vi "Begin.vi"() -> (0 "error out":errorcluster)   [LabVIEW 2013]
doc: "Called before other user functions, this VI is expected to open initial I/O refnums, load in file data, and do all program initialization. Notice that the <B>error out</B> terminal is simply used for data flow. Wiring it to other structures or subVIs ensures that this VI runs first."
uses:
  <vilib>/Rock Robotics/WPI/Joystick/WPI_JoystickDeviceEnum.ctl
  <vilib>/Rock Robotics/SystemInterfaces/Typedef/FPGA_TypedefDigitalModule.ctl
  <vilib>/Rock Robotics/SystemInterfaces/DIO/FPGA_DIOChannel.ctl
  <vilib>/Rock Robotics/SystemInterfaces/DIO/FPGA_DIORelayChannel.ctl
  <vilib>/Rock Robotics/SystemInterfaces/Typedef/FPGA_TypedefSolenoidModule.ctl
  <vilib>/Rock Robotics/WPI/Solenoid/WPI_SolenoidChannel.ctl
  <vilib>/Rock Robotics/SystemInterfaces/DIO/FPGA_DIOPWMChannel.ctl
  <vilib>/Rock Robotics/WPI/Encoder/WPI_EncoderType.ctl
  <vilib>/Rock Robotics/WPI/Solenoid/WPI_SolenoidValue.ctl
  <vilib>/Rock Robotics/SystemInterfaces/Typedef/FPGA_TypedefAnalogModule.ctl
  <vilib>/Rock Robotics/SystemInterfaces/AI/FPGA_AIChannel.ctl
  <vilib>/Rock Robotics/WPI/Solenoid/WPI_SolenoidOpenDouble.vi
  <vilib>/Rock Robotics/WPI/Solenoid/WPI_SolenoidSetEnum.vi
  <vilib>/Rock Robotics/WPI/Counter/WPI_CounterDigitalInputToDigitalSource.vi
  <vilib>/Rock Robotics/WPI/MotorControl/WPI_MotorControlOpen Jaguar.vi
  <vilib>/Rock Robotics/WPI/MotorControl/WPI_MotorControlOpen Victor.vi
  <vilib>/Rock Robotics/WPI/RobotDrive/WPI_RobotDriveOpen2MotorWithVictor.vi
  <vilib>/Rock Robotics/WPI/Compressor/WPI_CompressorGetSetRefNum.vi
  <vilib>/Rock Robotics/WPI/Camera/WPI_CameraImageSize.ctl
  <vilib>/Rock Robotics/WPI/Camera/WPI_CameraWhite Balance Values.ctl
  <vilib>/Rock Robotics/WPI/Camera/WPI_CameraExposure Values.ctl
  <vilib>/Rock Robotics/WPI/Camera/WPI_CameraFrameRate.ctl
  <vilib>/Rock Robotics/WPI/RobotDrive/WPI_RobotDriveOpen4MotorWithVictor.vi
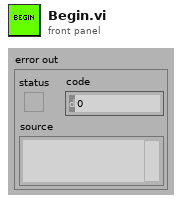
[diagram p1: front panel]
types:
  T1 = typedef "WPI_SolenoidValue.ctl" = enum16{"Off", "On", "Forward", "Reverse"}
  T2 = typedef "FPGA_AIChannel.ctl" = enum8{"AI 1", "AI 2", "AI 3", "AI 4", "AI 5", "AI 6", "AI 7", "AI 8", "Invalid"}
  T3 = typedef "FPGA_TypedefAnalogModule.ctl" = enum16{"Analog Module 1", "Analog Module 2"}
  T4 = typedef "FPGA_DIOChannel.ctl" = enum8{"DIO 1", "DIO 2", "DIO 3", "DIO 4", "DIO 5", "DIO 6", "DIO 7", "DIO 8", "DIO 9", "DIO 10", "DIO 11", "DIO 12", "DIO 13", "DIO 14", "Invalid"}
  T5 = typedef "WPI_SolenoidChannel.ctl" = enum8{"Solenoid 1", "Solenoid 2", "Solenoid 3", "Solenoid 4", "Solenoid 5", "Solenoid 6", "Solenoid 7", "Solenoid 8", "Invalid"}
  T6 = typedef "FPGA_DIOPWMChannel.ctl" = enum8{"PWM 1", "PWM 2", "PWM 3", "PWM 4", "PWM 5", "PWM 6", "PWM 7", "PWM 8", "PWM 9", "PWM 10", "Invalid"}
  T7 = typedef "WPI_EncoderType.ctl" = enum16{"1x", "2x", "4x"}
  T8 = typedef "FPGA_TypedefSolenoidModule.ctl" = enum16{"Solenoid Module 1", "Solenoid Module 2"}
  T9 = typedef "FPGA_DIORelayChannel.ctl" = enum8{"Relay 1", "Relay 2", "Relay 3", "Relay 4", "Relay 5", "Relay 6", "Relay 7", "Relay 8", "Invalid"}
  T10 = typedef "WPI_JoystickDeviceEnum.ctl" = enum16{"USB 1", "USB 2", "USB 3", "USB 4", "Kinect 1", "Kinect 2"}
  T11 = typedef "FPGA_TypedefDigitalModule.ctl" = enum16{"Digital Module 1", "Digital Module 2"}
  T12 = typedef "WPI_CameraFrameRate.ctl" = u32
  T13 = typedef "WPI_CameraExposure Values.ctl" = enum16{"Auto", "Flicker-free 50 Hz", "Flicker-free 60 Hz", "Hold current"}
  T14 = typedef "WPI_CameraWhite Balance Values.ctl" = enum16{"Auto", "Fixed indoor", "Fixed outdoor 1", "Fixed outdoor 2", "Fixed fluorescent 1", "Fixed fluorescent 2", "Hold current"}
  T15 = typedef "WPI_CameraImageSize.ctl" = enum16{"640x480", "320x240", "160x120"}
  T16 = typedef "WPI_CameraDevRef.ctl" = cluster{"Camera Address":string, "CameraStatus":errorcluster, "Acquire Image Notifier":refnum<notifier>}
  T17 = typedef "WPI_DigitalInputDevRef.ctl" = cluster{"DevStatus":errorcluster, "DIO Channel":T4, "Digital Module":T11}
  T18 = typedef "WPI_AnalogChannelDevRef.ctl" = cluster{"DevStatus":errorcluster, "Analog Module":T3, "Analog Channel":T2}
  T19 = typedef "WPI_RobotDriveDevRef.ctl" = cluster{"DevStatus":errorcluster, "Motors[]":T20[], "Square Inputs":bool, "Max Output":dbl, "Isochronous":bool}
  T20 = typedef "WPI_MotorControlDeviceRef.ctl" = cluster{"DeviceStatus":errorcluster, "Type":enum16{"PWM", "CAN"}, "PWM":cluster{"Digital Module":T11, "PWM Channel":T6, "DeadBand":T21}, "CAN":cluster{"Device Number":u8, "Control Mode":T22, "Semaphore":T23, "Max Vout":dbl}, "Invert":bool, "TransformRef":T24, "InvTransformRef":T24}
  T21 = typedef "WPI_PWMDeadband.ctl" = cluster{"Name":string, "maxPositivePwm":i32, "minPositivePwm":i32, "centerPwm":i32, "maxNegativePwm":i32, "minNegativePwm":i32, "angularRange":u16}
  T22 = typedef "WPI_CANJaguar_ControlMode.ctl" = enum8{"Percent VBus", "Current", "Speed", "Position", "Voltage"}
  T23 = typedef "Semaphore RefNum" = refnum<k1>
  T24 = typedef "WPI_PWMTransform_ConPane.ctl" = refnum<vi>
  T25 = typedef "WPI_SolenoidDevRef.ctl" = cluster{"DevStatus":errorcluster, "Solenoid Module":T8, "Forward Solenoid Channel":T5, "Reverse Solenoid Channel":T5}
  T26 = typedef "FPGA_CounterEncoderSourceConvertionLVSourceType.ctl" = cluster{"DevStatus":errorcluster, "AnalogTriggerMode?":bool, "DigitalMode":cluster{"Digital Module":T11, "DIO Channel":T27}, "AnalogTriggerMode":cluster{"AnalogTriggerIndex":T28, "OutputType":T29}}
  T27 = typedef "FPGA_DIODigitalSourceChannel.ctl" = enum8{"DIO 1", "DIO 2", "DIO 3", "DIO 4", "DIO 5", "DIO 6", "DIO 7", "DIO 8", "DIO 9", "DIO 10", "DIO 11", "DIO 12", "DIO 13", "DIO 14", "Disabled"}
  T28 = typedef "FPGA_AnalogTriggerIndex.ctl" = enum8{"Trig 0", "Trig 1", "Trig 2", "Trig 3", "Trig 4", "Trig 5", "Trig 6", "Trig 7", "Invalid"}
  T29 = typedef "FPGA_AnalogTriggerOutType.ctl" = enum16{"InWindow", "TriggerState", "Rising", "Falling"}
  T30 = typedef "WPI_CompressorDevRef.ctl" = cluster{"DevStatus":errorcluster, "DigitalInputDevRef":T17, "RelayDevRef":T31}
  T31 = typedef "WPI_RelayDevRef.ctl" = cluster{"DevStatus":errorcluster, "Relay Channel":T9, "Digital Module":T11, "Relay Direction":T32}
  T32 = typedef "WPI_RelayDirection.ctl" = enum16{"Both directions", "Forward only", "Reverse only"}
  T33 = typedef "WPI_EncoderDevRef.ctl" = cluster{"DevStatus":errorcluster, "EncoderIndex":T34, "CounterIndex":T35, "DistancePerCount":dbl, "Decoding Type":T7}
  T34 = typedef "FPGA_EncoderIdx.ctl" = enum8{"Enc 0", "Enc 1", "Enc 2", "Enc 3", "Invalid"}
  T35 = typedef "FPGA_CounterCtrSystemIndex.ctl" = enum8{"Ctr 0", "Ctr 1", "Ctr 2", "Ctr 3", "Ctr 4", "Ctr 5", "Ctr 6", "Ctr 7", "Invalid"}
  T36 = typedef "WPI_JoystickDevRef.ctl" = cluster{"Device":T10}
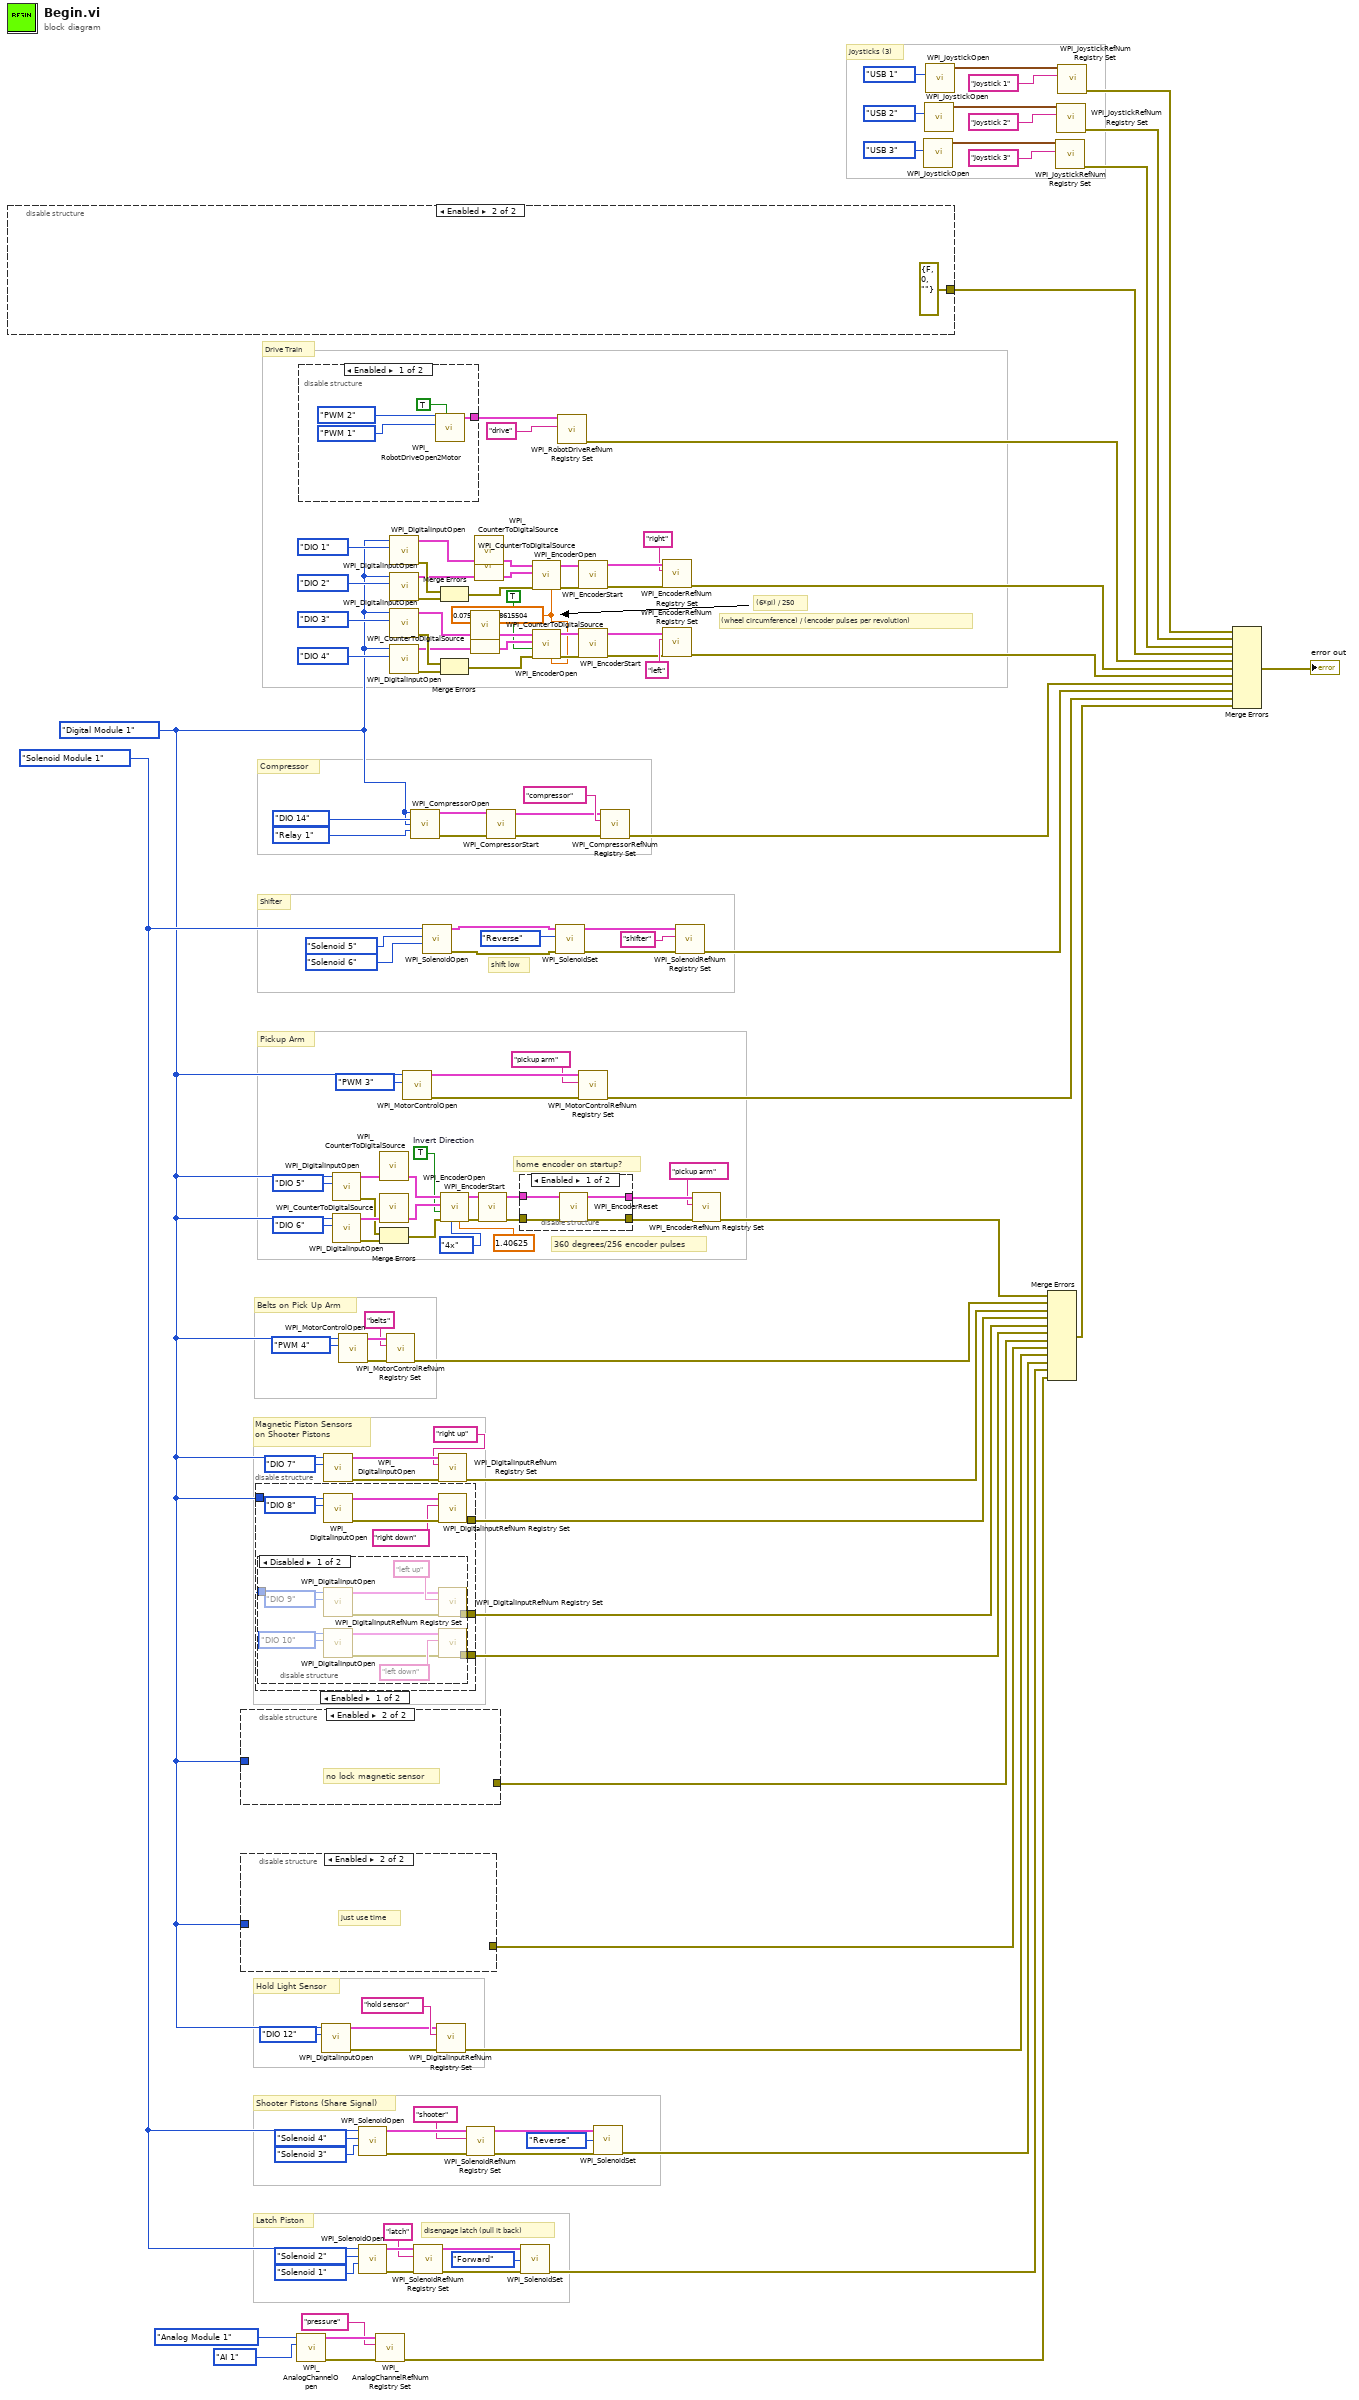
[diagram p0: block diagram]
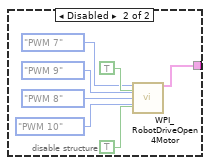
[diagram p2: hidden frame]
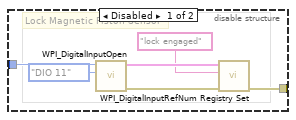
[diagram p3: hidden frame]
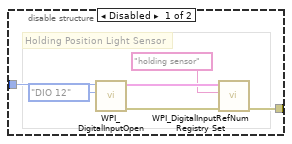
[diagram p6: hidden frame]
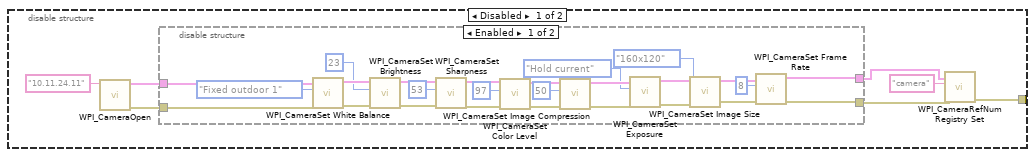
[diagram p8: hidden frame]
diagram:
  w13 = TRUE  # Invert Direction
  w84 = 0.07539822368615504 ("DistancePerCount")
  w27 = FPGA_TypedefSolenoidModule."Solenoid Module 1" ("Solenoid Module (Module 1)")
  w20 = FPGA_TypedefDigitalModule."Digital Module 1" ("Digital Module (Module 1)")
  # "360 degrees/256 encoder pulses"
  # "disengage latch (pull it back)"
  # "Hold Light Sensor"
  # "Joysticks (3)"
  # "Latch Piston"
  # "Shooter Pistons (Share Signal)"
  # "Magnetic Piston Sensors\non Shooter Pistons"
  # "Belts on Pick Up Arm"
  # "Pickup Arm"
  # "home encoder on startup?"
  # "Shifter"
  # "Compressor"
  # "Drive Train"
  # "shift low"
  # "(wheel circumference) / (encoder pulses per revolution)"
  # "(6*pi) / 250"
  n1 = disable-structure shown="Enabled" {
    disable-tunnel: [w139 errorcluster {"status"=FALSE, "code"=0, "source"=""} ("error out")] -> w126
    frame Disabled {
      n2 = call <vilib>:"WPI_CameraOpen.vi"("Camera Address"="10.11.24.11") -> ("error out"=w141:errorcluster, "CameraDevRef"=w143:T16)  [unwired: 9 in]
      n3 = disable-structure shown="Enabled" {
        disable-tunnel: w143 -> [w169 w173]
        disable-tunnel: [w147 w173] -> w142
        disable-tunnel: w141 -> [w156 w172]
        disable-tunnel: [w146 w172] -> w140
        frame Enabled {
          n4 = call <vilib>:"WPI_CameraSet White Balance.vi"("error in (no error)"=w156, "White Balance"=WPI_CameraWhite_Balance_Values."Fixed outdoor 1", "CameraDevRef"=w169) -> ("error out"=w157:errorcluster, "CameraDevRef Out"=w168:T16)  [unwired: 7 in]
          n5 = call <vilib>:"WPI_CameraSet Brightness.vi"("error in (no error)"=w157, "Brightness"=23, "CameraDevRef"=w168) -> ("error out"=w158:errorcluster, "CameraDevRef Out"=w167:T16)  [unwired: 7 in]
          n6 = call <vilib>:"WPI_CameraSet Sharpness.vi"("error in (no error)"=w158, "Sharpness"=53, "CameraDevRef"=w167) -> ("error out"=w159:errorcluster, "CameraDevRef Out"=w166:T16)  [unwired: 7 in]
          n7 = call <vilib>:"WPI_CameraSet Color Level.vi"("error in (no error)"=w159, "Color Level"=97, "CameraDevRef"=w166) -> ("error out"=w160:errorcluster, "CameraDevRef Out"=w165:T16)  [unwired: 7 in]
          n8 = call <vilib>:"WPI_CameraSet Image Compression.vi"("error in (no error)"=w160, "Compression"=50, "CameraDevRef"=w165) -> ("error out"=w171:errorcluster, "CameraDevRef Out"=w170:T16)  [unwired: 7 in]
          n9 = call <vilib>:"WPI_CameraSet Exposure.vi"("error in (no error)"=w171, "Exposure"=WPI_CameraExposure_Values."Hold current", "CameraDevRef"=w170) -> ("error out"=w161:errorcluster, "CameraDevRef Out"=w164:T16)  [unwired: 7 in]
          n10 = call <vilib>:"WPI_CameraSet Image Size.vi"("error in (no error)"=w161, "Image Size"=WPI_CameraImageSize."160x120", "CameraDevRef"=w164) -> ("error out"=w162:errorcluster, "CameraDevRef Out"=w163:T16)  [unwired: 7 in]
          n11 = call <vilib>:"WPI_CameraSet Frame Rate.vi"("error in (no error)"=w162, "Frame Rate (fps)"=T12 8, "CameraDevRef"=w163) -> ("error out"=w146:errorcluster, "CameraDevRef Out"=w147:T16)  [unwired: 7 in]
        }
        frame Disabled {
        }
      }
      n12 = call <vilib>:"WPI_CameraRefNum Registry Set.vi"("error in (no error)"=w140, "refnum name"="camera", "CameraDevRef"=w142) -> ("error out"=w139:errorcluster)  [unwired: 7 in, 1 out]
    }
    frame Enabled {
    }
  }
  n13 = disable-structure shown="Enabled" {
    disable-tunnel: w20 -> [w176 _]
    disable-tunnel: [w175 _] -> w17
    frame Disabled {
      # "Lock Magnetic Piston Sensor"
      n14 = call <vilib>:"WPI_DigitalInputOpen.vi"("DIO Channel"=FPGA_DIOChannel."DIO 11", "Digital Module (Module 1)"=w176) -> ("error out"=w179:errorcluster, "DigitalInputDevRef"=w178:T17)  [unwired: 8 in]
      n15 = call <vilib>:"WPI_DigitalInputRefNum Registry Set.vi"("error in (no error)"=w179, "refnum name"="lock engaged", "DigitalInputDevRef"=w178) -> ("error out"=w175:errorcluster)  [unwired: 7 in, 1 out]
    }
    frame Enabled {
      # "no lock magnetic sensor"
    }
  }
  n16 = disable-structure shown="Enabled" {
    disable-tunnel: w20 -> [w182 _]
    disable-tunnel: [w181 _] -> w18
    frame Disabled {
      # "Holding Position Light Sensor"
      n17 = call <vilib>:"WPI_DigitalInputOpen.vi"("DIO Channel"=FPGA_DIOChannel."DIO 12", "Digital Module (Module 1)"=w182) -> ("error out"=w185:errorcluster, "DigitalInputDevRef"=w184:T17)  [unwired: 8 in]
      n18 = call <vilib>:"WPI_DigitalInputRefNum Registry Set.vi"("error in (no error)"=w185, "refnum name"="holding sensor", "DigitalInputDevRef"=w184) -> ("error out"=w181:errorcluster)  [unwired: 7 in, 1 out]
    }
    frame Enabled {
      # "just use time"
    }
  }
  n19 = disable-structure shown="Enabled" {
    disable-tunnel: [w191 _] -> w38
    disable-tunnel: w20 -> [w189 _]
    disable-tunnel: [w188 _] -> w22
    disable-tunnel: [w187 _] -> w21
    frame Enabled {
      n20 = disable-structure shown="Disabled" {
        disable-tunnel: w189 -> [w197 _]
        disable-tunnel: [w196 _] -> w188
        disable-tunnel: [w195 _] -> w187
        frame Disabled {
          n21 = call <vilib>:"WPI_DigitalInputOpen.vi"("DIO Channel"=FPGA_DIOChannel."DIO 9", "Digital Module (Module 1)"=w197) -> ("error out"=w198:errorcluster, "DigitalInputDevRef"=w199:T17)  [unwired: 8 in]
          n22 = call <vilib>:"WPI_DigitalInputOpen.vi"("DIO Channel"=FPGA_DIOChannel."DIO 10", "Digital Module (Module 1)"=w197) -> ("error out"=w200:errorcluster, "DigitalInputDevRef"=w201:T17)  [unwired: 8 in]
          n23 = call <vilib>:"WPI_DigitalInputRefNum Registry Set.vi"("error in (no error)"=w198, "refnum name"="left up", "DigitalInputDevRef"=w199) -> ("error out"=w196:errorcluster)  [unwired: 7 in, 1 out]
          n24 = call <vilib>:"WPI_DigitalInputRefNum Registry Set.vi"("error in (no error)"=w200, "refnum name"="left down", "DigitalInputDevRef"=w201) -> ("error out"=w195:errorcluster)  [unwired: 7 in, 1 out]
        }
        frame Enabled {
        }
      }
      n25 = call <vilib>:"WPI_DigitalInputOpen.vi"("DIO Channel"=FPGA_DIOChannel."DIO 8", "Digital Module (Module 1)"=w189) -> ("error out"=w194:errorcluster, "DigitalInputDevRef"=w193:T17)  [unwired: 8 in]
      n26 = call <vilib>:"WPI_DigitalInputRefNum Registry Set.vi"("error in (no error)"=w194, "refnum name"="right down", "DigitalInputDevRef"=w193) -> ("error out"=w191:errorcluster)  [unwired: 7 in, 1 out]
    }
    frame Disabled {
      # "dang, only one sensor\non the pistons..."
    }
  }
  n27 = call <vilib>:"WPI_AnalogChannelOpen.vi"("Analog Channel"=FPGA_AIChannel."AI 1", "Analog Module (Module 1)"=FPGA_TypedefAnalogModule."Analog Module 1") -> ("error out"=w10:errorcluster, "AIDeviceRef"=w9:T18)  [unwired: 8 in]
  n28 = disable-structure shown="Enabled" {
    disable-tunnel: [w209 w216] -> w106
    frame Enabled {
      n29 = call-poly <vilib>:"WPI_RobotDriveOpen2Motor.vi"("Left Motor Inverted"=TRUE, "Right Motor"=FPGA_DIOPWMChannel."PWM 1", "Left Motor"=FPGA_DIOPWMChannel."PWM 2") -> ("RobotDriveDevRef"=w209:T19)  [unwired: 7 in, 1 out]
    }
    frame Disabled {
      n30 = call-poly <vilib>:"WPI_RobotDriveOpen4Motor.vi"("Rear Left Motor"=FPGA_DIOPWMChannel."PWM 7", "Rear Left Motor Inverted"=TRUE, "Rear Right Motor"=FPGA_DIOPWMChannel."PWM 9", "Front Left Motor"=FPGA_DIOPWMChannel."PWM 8", "Front Right Motor"=FPGA_DIOPWMChannel."PWM 10", "Front Left Motor Inverted"=TRUE) -> ("RobotDriveDevRef"=w216:T19)  [unwired: 8 in, 1 out]
    }
  }
  n31 = call <vilib>:"WPI_DigitalInputOpen.vi"("DIO Channel"=FPGA_DIOChannel."DIO 12", "Digital Module (Module 1)"=w20) -> ("error out"=w24:errorcluster, "DigitalInputDevRef"=w25:T17)  [unwired: 8 in]
  n32 = call <vilib>:"WPI_DigitalInputOpen.vi"("DIO Channel"=FPGA_DIOChannel."DIO 7", "Digital Module (Module 1)"=w20) -> ("error out"=w43:errorcluster, "DigitalInputDevRef"=w42:T17)  [unwired: 8 in]
  n33 = call <vilib>:"WPI_DigitalInputOpen.vi"("DIO Channel"=FPGA_DIOChannel."DIO 5", "Digital Module (Module 1)"=w20) -> ("error out"=w61:errorcluster, "DigitalInputDevRef"=w66:T17)  [unwired: 8 in]
  n34 = call <vilib>:"WPI_DigitalInputOpen.vi"("DIO Channel"=FPGA_DIOChannel."DIO 6", "Digital Module (Module 1)"=w20) -> ("error out"=w62:errorcluster, "DigitalInputDevRef"=w65:T17)  [unwired: 8 in]
  n35 = call-poly <vilib>:"WPI_MotorControlOpen.vi"("PWM Channel"=FPGA_DIOPWMChannel."PWM 4", "Digital Module (Module 1)"=w20) -> ("error out"=w49:errorcluster, "MotorControlDeviceRef"=w48:T20)  [unwired: 8 in]
  n36 = call-poly <vilib>:"WPI_SolenoidOpen.vi"("Reverse Solenoid Channel"=WPI_SolenoidChannel."Solenoid 3", "Forward Solenoid Channel"=WPI_SolenoidChannel."Solenoid 4", "Solenoid Module (Module 1)"=w27) -> ("error out"=w33:errorcluster, "SolenoidDevRef"=w32:T25)  [unwired: 7 in]
  n37 = call-poly <vilib>:"WPI_SolenoidOpen.vi"("Reverse Solenoid Channel"=WPI_SolenoidChannel."Solenoid 1", "Forward Solenoid Channel"=WPI_SolenoidChannel."Solenoid 2", "Solenoid Module (Module 1)"=w27) -> ("error out"=w31:errorcluster, "SolenoidDevRef"=w30:T25)  [unwired: 7 in]
  n38 = call <vilib>:"WPI_AnalogChannelRefNum Registry Set.vi"("error in (no error)"=w10, "refnum name"="pressure", "AIDeviceRef"=w9) -> ("error out"=w7:errorcluster)  [unwired: 7 in, 1 out]
  n39 = call-poly <vilib>:"WPI_CounterToDigitalSource.vi"("DigitalInputDevRef"=w66) -> ("Digital Source"=w64:T26)  [unwired: 6 in]
  n40 = call-poly <vilib>:"WPI_CounterToDigitalSource.vi"("DigitalInputDevRef"=w65) -> ("Digital Source"=w63:T26)  [unwired: 6 in]
  n41 = Merge Errors(w61, w62) -> (w60:errorcluster)
  n42 = call <vilib>:"WPI_MotorControlRefNum Registry Set.vi"("error in (no error)"=w49, "refnum name"="belts", "MotorControlDevRef"=w48) -> ("error out"=w46:errorcluster)  [unwired: 7 in, 1 out]
  n43 = call <vilib>:"WPI_DigitalInputOpen.vi"("DIO Channel"=FPGA_DIOChannel."DIO 1", "Digital Module (Module 1)"=w20) -> ("error out"=w78:errorcluster, "DigitalInputDevRef"=w90:T17)  [unwired: 8 in]
  n44 = call <vilib>:"WPI_DigitalInputOpen.vi"("DIO Channel"=FPGA_DIOChannel."DIO 2", "Digital Module (Module 1)"=w20) -> ("error out"=w80:errorcluster, "DigitalInputDevRef"=w77:T17)  [unwired: 8 in]
  n45 = call <vilib>:"WPI_DigitalInputOpen.vi"("DIO Channel"=FPGA_DIOChannel."DIO 3", "Digital Module (Module 1)"=w20) -> ("error out"=w81:errorcluster, "DigitalInputDevRef"=w104:T17)  [unwired: 8 in]
  n46 = call <vilib>:"WPI_DigitalInputOpen.vi"("DIO Channel"=FPGA_DIOChannel."DIO 4", "Digital Module (Module 1)"=w20) -> ("error out"=w83:errorcluster, "DigitalInputDevRef"=w76:T17)  [unwired: 8 in]
  n47 = call-poly <vilib>:"WPI_MotorControlOpen.vi"("PWM Channel"=FPGA_DIOPWMChannel."PWM 3", "Digital Module (Module 1)"=w20) -> ("error out"=w73:errorcluster, "MotorControlDeviceRef"=w72:T20)  [unwired: 8 in]
  n48 = call <vilib>:"WPI_CompressorOpen.vi"("Pressure Switch Digital Module (Module 1)"=w20, "Pressure Switch DIO Channel"=FPGA_DIOChannel."DIO 14", "Relay Digital Module (Module 1)"=w20, "Relay Channel"=FPGA_DIORelayChannel."Relay 1") -> ("CompressorDevRef"=w118:T30, "error out"=w117:errorcluster)  [unwired: 10 in]
  n49 = call <vilib>:"WPI_SolenoidRefNum Registry Set.vi"("error in (no error)"=w31, "refnum name"="latch", "SolenoidDevRef"=w30) -> ("error out"=w16:errorcluster, "SolenoidDevRef"=w15:T25)  [unwired: 7 in]
  n50 = call-poly <vilib>:"WPI_SolenoidOpen.vi"("Reverse Solenoid Channel"=WPI_SolenoidChannel."Solenoid 6", "Forward Solenoid Channel"=WPI_SolenoidChannel."Solenoid 5", "Solenoid Module (Module 1)"=w27) -> ("error out"=w109:errorcluster, "SolenoidDevRef"=w110:T25)  [unwired: 7 in]
  n51 = call <vilib>:"WPI_DigitalInputRefNum Registry Set.vi"("error in (no error)"=w24, "refnum name"="hold sensor", "DigitalInputDevRef"=w25) -> ("error out"=w19:errorcluster)  [unwired: 7 in, 1 out]
  n52 = call <vilib>:"WPI_DigitalInputRefNum Registry Set.vi"("error in (no error)"=w43, "refnum name"="right up", "DigitalInputDevRef"=w42) -> ("error out"=w39:errorcluster)  [unwired: 7 in, 1 out]
  n53 = Merge Errors(w78, w80) -> (w79:errorcluster)
  n54 = Merge Errors(w81, w83) -> (w82:errorcluster)
  n55 = call <vilib>:"WPI_EncoderOpen.vi"("DistancePerCount"=1.40625, "Decoding Type"=WPI_EncoderType."4x", "error in (no error)"=w60, "Invert Direction (False)"=w13, "BSource"=w63, "ASource"=w64) -> ("error out"=w59:errorcluster, "EncoderDevRef"=w58:T33)  [unwired: 4 in]
  n56 = call <vilib>:"WPI_SolenoidRefNum Registry Set.vi"("error in (no error)"=w33, "refnum name"="shooter", "SolenoidDevRef"=w32) -> ("error out"=w4:errorcluster, "SolenoidDevRef"=w3:T25)  [unwired: 7 in]
  n57 = call-poly <vilib>:"WPI_CounterToDigitalSource.vi"("DigitalInputDevRef"=w104) -> ("Digital Source"=w97:T26)  [unwired: 6 in]
  n58 = call-poly <vilib>:"WPI_CounterToDigitalSource.vi"("DigitalInputDevRef"=w76) -> ("Digital Source"=w98:T26)  [unwired: 6 in]
  n59 = call-poly <vilib>:"WPI_CounterToDigitalSource.vi"("DigitalInputDevRef"=w90) -> ("Digital Source"=w96:T26)  [unwired: 6 in]
  n60 = call-poly <vilib>:"WPI_CounterToDigitalSource.vi"("DigitalInputDevRef"=w77) -> ("Digital Source"=w95:T26)  [unwired: 6 in]
  n61 = call <vilib>:"WPI_EncoderStart.vi"("error in (no error)"=w59, "EncoderDevRef"=w58) -> ("error out"=w57:errorcluster, "EncoderDevRef"=w56:T33)  [unwired: 8 in]
  n62 = call <vilib>:"WPI_CompressorStart.vi"("error in (no error)"=w117, "CompressorDevRef"=w118) -> ("error out"=w116:errorcluster, "CompressorDevRef"=w115:T30)  [unwired: 8 in]
  n63 = disable-structure shown="Enabled" {
    disable-tunnel: w57 -> [w220 w221]
    disable-tunnel: w56 -> [w219 w222]
    disable-tunnel: [w218 w222] -> w54
    disable-tunnel: [w217 w221] -> w55
    frame Enabled {
      n64 = call <vilib>:"WPI_EncoderReset.vi"("error in (no error)"=w220, "EncoderDevRef"=w219) -> ("error out"=w217:errorcluster, "EncoderDevRef"=w218:T33)  [unwired: 8 in]
    }
    frame Disabled {
    }
  }
  n65 = call-poly <vilib>:"WPI_SolenoidSet.vi"("error in (no error)"=w16, "Value"=WPI_SolenoidValue."Forward", "SolenoidDevRef"=w15) -> ("error out"=w6:errorcluster)  [unwired: 7 in, 1 out]
  n66 = call <vilib>:"WPI_EncoderOpen.vi"("DistancePerCount"=w84, "error in (no error)"=w79, "BSource"=w95, "ASource"=w96) -> ("error out"=w94:errorcluster, "EncoderDevRef"=w93:T33)  [unwired: 6 in]
  n67 = call <vilib>:"WPI_EncoderOpen.vi"("DistancePerCount"=w84, "error in (no error)"=w82, "Invert Direction (False)"=TRUE, "BSource"=w98, "ASource"=w97) -> ("error out"=w99:errorcluster, "EncoderDevRef"=w100:T33)  [unwired: 5 in]
  n68 = call-poly <vilib>:"WPI_SolenoidSet.vi"("error in (no error)"=w109, "Value"=WPI_SolenoidValue."Reverse", "SolenoidDevRef"=w110) -> ("error out"=w108:errorcluster, "SolenoidDevRef"=w107:T25)  [unwired: 7 in]
  n69 = call <vilib>:"WPI_RobotDriveRefNum Registry Set.vi"("refnum name"="drive", "RobotDriveDevRef"=w106) -> ("error out"=w125:errorcluster)  [unwired: 8 in, 1 out]
  n70 = call <vilib>:"WPI_EncoderStart.vi"("error in (no error)"=w94, "EncoderDevRef"=w93) -> ("error out"=w92:errorcluster, "EncoderDevRef"=w91:T33)  [unwired: 8 in]
  n71 = call <vilib>:"WPI_EncoderStart.vi"("error in (no error)"=w99, "EncoderDevRef"=w100) -> ("error out"=w101:errorcluster, "EncoderDevRef"=w102:T33)  [unwired: 8 in]
  n72 = call <vilib>:"WPI_MotorControlRefNum Registry Set.vi"("error in (no error)"=w73, "refnum name"="pickup arm", "MotorControlDevRef"=w72) -> ("error out"=w69:errorcluster)  [unwired: 7 in, 1 out]
  n73 = call-poly <vilib>:"WPI_SolenoidSet.vi"("error in (no error)"=w4, "Value"=WPI_SolenoidValue."Reverse", "SolenoidDevRef"=w3) -> ("error out"=w2:errorcluster)  [unwired: 7 in, 1 out]
  n74 = call <vilib>:"WPI_CompressorRefNum Registry Set.vi"("error in (no error)"=w116, "refnum name"="compressor", "CompressorDevRef"=w115) -> ("error out"=w74:errorcluster)  [unwired: 7 in, 1 out]
  n75 = call <vilib>:"WPI_EncoderRefNum Registry Set.vi"("error in (no error)"=w92, "refnum name"="right", "EncoderDevRef"=w91) -> ("error out"=w124:errorcluster)  [unwired: 7 in, 1 out]
  n76 = call <vilib>:"WPI_EncoderRefNum Registry Set.vi"("error in (no error)"=w101, "refnum name"="left", "EncoderDevRef"=w102) -> ("error out"=w123:errorcluster)  [unwired: 7 in, 1 out]
  n77 = call <vilib>:"WPI_SolenoidRefNum Registry Set.vi"("error in (no error)"=w108, "refnum name"="shifter", "SolenoidDevRef"=w107) -> ("error out"=w75:errorcluster)  [unwired: 7 in, 1 out]
  n78 = call <vilib>:"WPI_EncoderRefNum Registry Set.vi"("error in (no error)"=w55, "refnum name"="pickup arm", "EncoderDevRef"=w54) -> ("error out"=w45:errorcluster)  [unwired: 7 in, 1 out]
  n79 = call <vilib>:"WPI_JoystickOpen.vi"("JoystickDevice"=WPI_JoystickDeviceEnum."USB 3") -> ("JoystickDevRef"=w137:T36)  [unwired: 10 in]
  n80 = call <vilib>:"WPI_JoystickOpen.vi"("JoystickDevice"=WPI_JoystickDeviceEnum."USB 2") -> ("JoystickDevRef"=w134:T36)  [unwired: 10 in]
  n81 = call <vilib>:"WPI_JoystickOpen.vi"("JoystickDevice"=WPI_JoystickDeviceEnum."USB 1") -> ("JoystickDevRef"=w131:T36)  [unwired: 10 in]
  n82 = Merge Errors(w45, w46, w39, w38, w22, w21, w17, w18, w19, w2, w6, w7) -> (w44:errorcluster)
  n83 = call <vilib>:"WPI_JoystickRefNum Registry Set.vi"("refnum name"="Joystick 3", "JoystickDevRef"=w137) -> ("error out"=w127:errorcluster)  [unwired: 8 in, 1 out]
  n84 = call <vilib>:"WPI_JoystickRefNum Registry Set.vi"("refnum name"="Joystick 2", "JoystickDevRef"=w134) -> ("error out"=w128:errorcluster)  [unwired: 8 in, 1 out]
  n85 = call <vilib>:"WPI_JoystickRefNum Registry Set.vi"("refnum name"="Joystick 1", "JoystickDevRef"=w131) -> ("error out"=w129:errorcluster)  [unwired: 8 in, 1 out]
  n86 = Merge Errors(w129, w128, w127, w126, w125, w124, w123, w74, w75, w69, w44) -> (→"error out":errorcluster)
